vi "Get Tree Data.vi"(8 "error in":errorcluster, 9 "Headers":string[](array[string])=["Packet_Number", "Timestamp", "Source", "Destination", "Protocol", "Length", "Data"], 10 "Filter":refnum<vi>, 11 "Tree ref":refnum<vi>) -> (0 "error out":errorcluster, 3 "Array":string[][](array[string]))   [LabVIEW 2025, in "CAN-LIN Raw Bus Capture UI.lvlib"]
uses:
  CAN-LIN Raw Bus Capture UI.lvlib
  Table_Filtering/Table_Filtering.lvlib
panel:
  in  "Find element":string
  in  "Find Header":string
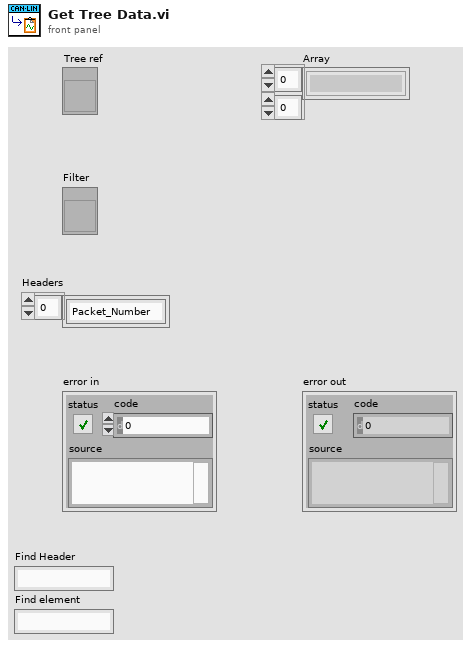
[diagram p1: front panel]
types:
  T1 = cluster{"FIELD":string, "OPERATOR":string, "VALUE":string}[]
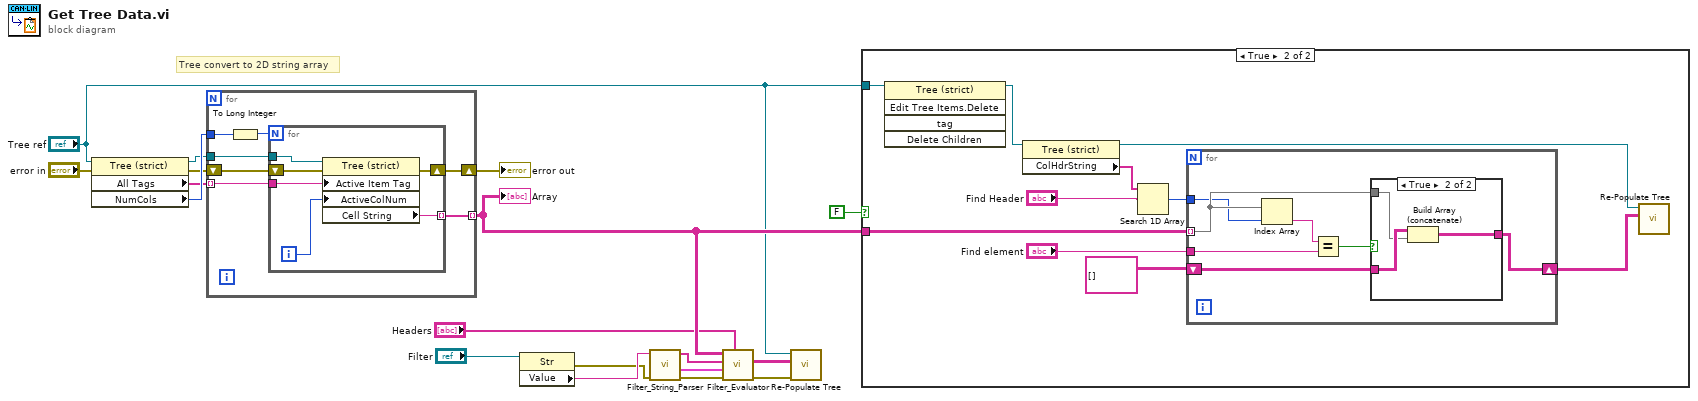
[diagram p0: block diagram]
diagram:
  # "Tree convert to 2D string array"
  n1 = property class="Tree (strict)"(reference="Tree ref", error in="error in") -> (reference out=w13:refnum<vi>, error out=w15:errorcluster, "All Tags"=w17:string[], "NumCols"=w18:u32)
  n2 = for {
    tunnel: w13 -> [w25]
    tunnel: w17 -> [w24] mode=indexing
    tunnel: w18 -> [w21]
    tunnel: [w23] -> w12 mode=indexing
    shift-right: [w19] -> w14
    shift-left: w15 -> [w20]
    n3 = To Long Integer(number=w21) -> (32bit integer=w22:i32)
    n4 = for {
      N: w22 -> [_]
      tunnel: w25 -> [w31]
      tunnel: w24 -> [w30]
      tunnel: [w28] -> w23 mode=indexing
      shift-right: [w26] -> w19
      shift-left: w20 -> [w27]
      i -> [w29]
      n5 = property class="Tree (strict)"(reference=w31, error in=w27, "Active Item Tag"=w30, "ActiveColNum"=w29) -> (error out=w26:errorcluster, "Cell String"=w28:string)  [unwired: 1 out]
    }
  }
  "Array" <- w12
  "error out" <- w14
  n6 = property class="Str"(reference="Filter") -> (error out=w1:errorcluster, "Value"=w2:string)  [unwired: 1 in, 1 out]
  n7 = call "Filter_String_Parser.vi"("error in"=w1, "Filter String"=w2) -> ("error constant"=w10:errorcluster, "Comparators"=w9:T1, "Boolean Connectors"=w8:string[])  [unwired: 7 in]
  n8 = call "Filter_Evaluator.vi"("Headers"="Headers", "Error"=w10, "Comparators"=w9, "Boolean Connectors"=w8, "Prefiltered Data"=w12) -> ("Error Out"=w6:errorcluster, "Filtered Array"=w7:string[][])  [unwired: 4 in, 1 out]
  n9 = call "Re-Populate Tree.vi"("error in"=w6, "Array"=w7, "TreeControl in"="Tree ref") -> ()  [unwired: 8 in, 1 out]
  n10 = case shown="True" FALSE {
    tunnel: w12 -> [_ w32]
    tunnel: "Tree ref" -> [_ w34]
    frame False {
    }
    frame True {
      n11 = invoke class="Tree (strict)" method="Edit Tree Items.Delete"(reference=w34) -> (reference out=w33:refnum<vi>)  [unwired: 4 in, 4 out]
      n12 = property class="Tree (strict)"(reference=w33) -> (reference out=w35:refnum<vi>, "ColHdrString"=w39:string[])  [unwired: 1 in, 1 out]
      n13 = Search 1D Array(1D array=w39, element="Find Header") -> (index of element=w37:i32)  [unwired: 1 in]
      n14 = for {
        tunnel: w32 -> [w47] mode=indexing
        shift-right: [w46] -> w41
        shift-left: string[][] [] -> [w45]
        tunnel: w37 -> [w44]
        tunnel: "Find element" -> [w42]
        n15 = Index Array(array=w47, index=w44) -> (element=w43:string)
        n16 = Equal?(x=w43, y=w42) -> (x = y?=w48:bool)
        n17 = case shown="True" w48 {
          tunnel: w47 -> [_ w50]
          tunnel: w45 -> [w49 w51]
          tunnel: [w49 w52] -> w46
          frame False {
          }
          frame True {
            n18 = Build Array (concatenate)(w51, w50) -> (w52:string[][])
          }
        }
      }
      n19 = call "Re-Populate Tree.vi"("Array"=w41, "TreeControl in"=w35) -> ()  [unwired: 9 in, 1 out]
    }
  }
